vi "Get DataType Description.vi"   [LabVIEW 2017]
doc: "Palette helper grouping the data type description VIs, which return a readable description and an MD5 hash for a data type."
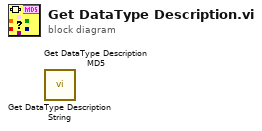
[diagram p0: block diagram]
diagram:
  n1 = call "Get DataType Description String.vi"() -> ()  [unwired: 10 in, 2 out]
  n2 = call "Get DataType Description MD5.vi"() -> ()  [unwired: 10 in, 2 out]
